vi "ORP_所有参数读取.vi"(8 "error in (no error)":errorcluster caption="错误输入（无错误）", 11 "MB session in":refnum<class "MB_Master.lvclass">) -> (0 "error out":errorcluster caption="错误输出", 2 "输出值":T1 {"电极型号标志" items=["NULL", "pH", "Cond", "DO", "Turb", "ORP"]; "电极状态标志" items=["OK"]}, 3 "MB session out":refnum<class "MB_Master.lvclass">)   [LabVIEW 2016, in "斯坦道多参数.lvlib"]
uses:
  <vilib>/Plasmionique/MB Master/MB_Master/MB_Master.lvclass
  <vilib>/Plasmionique/MB Master/MB Master.lvlib
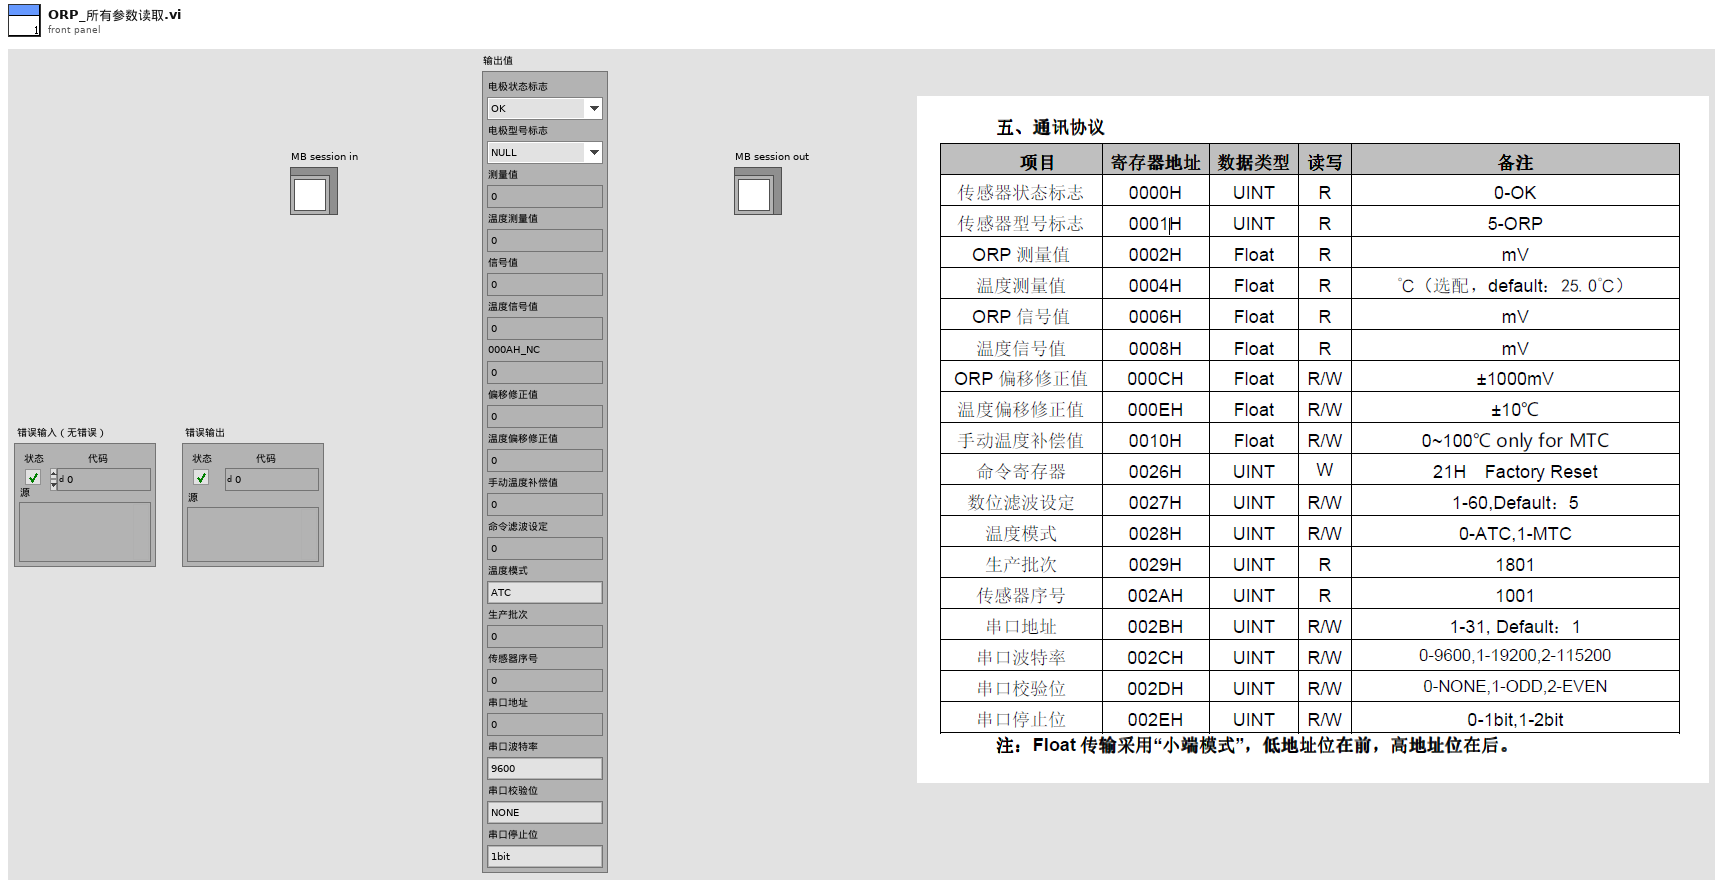
[diagram p1: front panel]
types:
  T1 = cluster{"电极状态标志":u16, "电极型号标志":u16, "测量值":sgl, "温度测量值":sgl, "信号值":sgl, "温度信号值":sgl, "000AH_NC":sgl, "偏移修正值":sgl, "温度偏移修正值":sgl, "手动温度补偿值":sgl, "命令滤波设定":u16, "温度模式":enum16{"ATC", "MTC"}, "生产批次":u16, "传感器序号":u16, "串口地址":u16, "串口波特率":enum16{"9600", "19200", "115200"}, "串口校验位":enum16{"NONE", "ODD", "EVEN"}, "串口停止位":enum16{"1bit", "2bit"}}
  T2 = cluster{u16, u16, "数值":sgl, "数值":sgl, "数值":sgl, "数值":sgl, "数值":sgl, "数值":sgl, "数值":sgl, "数值":sgl, u16, u16, u16, u16, u16, u16, u16, u16}
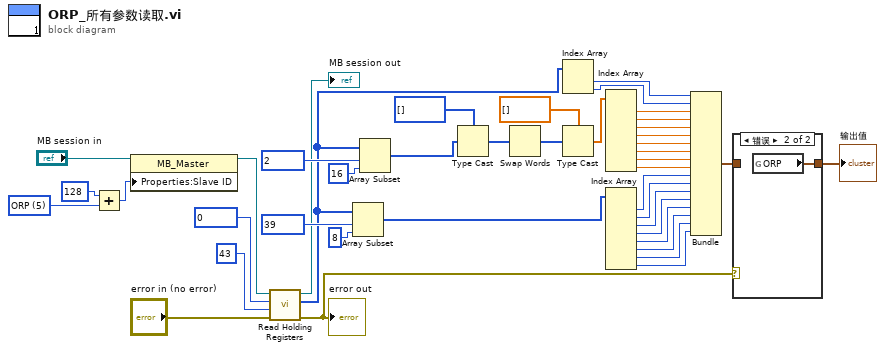
[diagram p0: block diagram]
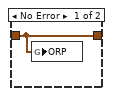
[diagram p2: hidden frame]
diagram:
  w42 = u16 5 items=["NULL", "pH", "Cond", "DO", "Turb", "ORP"] ("数值")
  n1 = Add(x=u16 128, y=w42) -> (x+y=w41:u16)
  n2 = property class="MB_Master"(reference="MB session in", "Properties:Slave ID"=w41) -> (reference out=w11:refnum<class "MB_Master.lvclass">)  [unwired: 1 in, 1 out]
  n3 = call <vilib>:"Read Holding Registers.vi"("error in (no error)"="error in (no error)", "quantity"=u16 43, "starting address"=u16 0, "MB session in"=w11) -> ("error out"=w7:errorcluster, "Registers"=w13:u16[], "MB session out"=→"MB session out":refnum<class "MB_Master.lvclass">)  [unwired: 5 in]
  "error out" <- w7
  n4 = Array Subset(array=w13, index=u16 39 ("starting address"), length=8 ("长度")) -> (w22:u16[])
  n5 = Array Subset(array=w13, index=u16 2 ("starting address"), length=16 ("长度")) -> (w30:u16[])
  n6 = Type Cast(type=u32[] [] ("数组 2"), x=w30) -> (*(type *) &x=w32:u32[])
  n7 = Swap Words(1:w32) -> (0:w34:u32[])
  n8 = Index Array(array=w13) -> (element #1=w37:u16, element #2=w36:u16)  [unwired: 2 in]
  n9 = Type Cast(type=sgl[] [] ("数组 2"), x=w34) -> (*(type *) &x=w29:sgl[])
  n10 = Index Array(array=w29) -> (element #1=w2:sgl, element #2=w28:sgl, element #3=w27:sgl, element #4=w26:sgl, element #5=w10:sgl, element #6=w9:sgl, element #7=w8:sgl, element #8=w4:sgl)  [unwired: 8 in]
  n11 = Index Array(array=w22) -> (element #1=w21:u16, element #2=w20:u16, element #3=w19:u16, element #4=w18:u16, element #5=w17:u16, element #6=w16:u16, element #7=w15:u16, element #8=w14:u16)  [unwired: 8 in]
  n12 = Bundle(w37, w36, "数值"=w2, "数值"=w28, "数值"=w27, "数值"=w26, "数值"=w10, "数值"=w9, "数值"=w8, "数值"=w4, w21, w20, w19, w18, w17, w16, w15, w14) -> (w3:T2)  [unwired: 1 in]
  n13 = case shown="错误" w7 {
    tunnel: w3 -> [w43 _]
    tunnel: [w43 w44] -> w1
    frame No Error {
      n14 = global write "国弘过程全局变量.vi" "ORP"(w43) -> ()
    }
    frame Error {
      n15 = global read "国弘过程全局变量.vi" "ORP"() -> (w44:T1)
    }
  }
  "输出值" <- w1
